vi "Fill List from DB (SubVI).vi"(4 "error in":errorcluster, 5 "ColumnName":string=" ", 7 "DropDownList":refnum<vi>) -> (0 "error out":errorcluster)   [LabVIEW 2010]
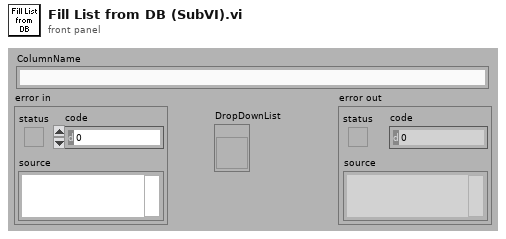
[diagram p1: front panel]
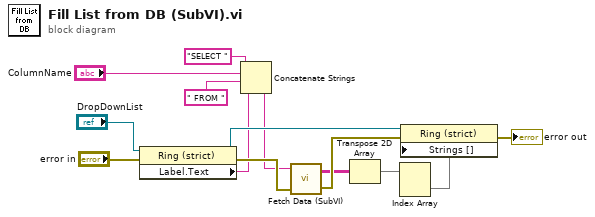
[diagram p0: block diagram]
diagram:
  n1 = property class="Ring (strict)"(reference="DropDownList", error in="error in") -> (reference out=w12:refnum<vi>, error out=w8:errorcluster, "Label.Text"=w2:string)
  n2 = Concatenate Strings("SELECT ", "ColumnName", " FROM ", w2) -> (w1:string)
  n3 = call "Fetch Data (SubVI).vi"("error IN"=w8, "query string"=w1) -> ("error OUT"=w7:errorcluster, "recordset data"=w6:string[][])  [unwired: 1 out]
  n4 = Transpose 2D Array(2D array=w6) -> (transposed array=w14:string[][])
  n5 = Index Array(array=w14) -> (element=w13:string[])  [unwired: 2 in]
  n6 = property class="Ring (strict)"(reference=w12, error in=w7, "Strings []"=w13) -> (error out=→"error out":errorcluster)  [unwired: 1 out]
